vi "Get Tables.vi"(8 "error in (no error)":errorcluster, 10 "System Tables (F)":bool, 11 "MS Access in":refnum<class "MS Access.lvclass">) -> (0 "error out":errorcluster, 2 "Table Names":string[](array[string]), 3 "MS Access out":refnum<class "MS Access.lvclass">)   [LabVIEW 2020, in "MS Access.lvclass"]
uses:
  MS Access.lvclass
  ODBC/ADODB.lvclass
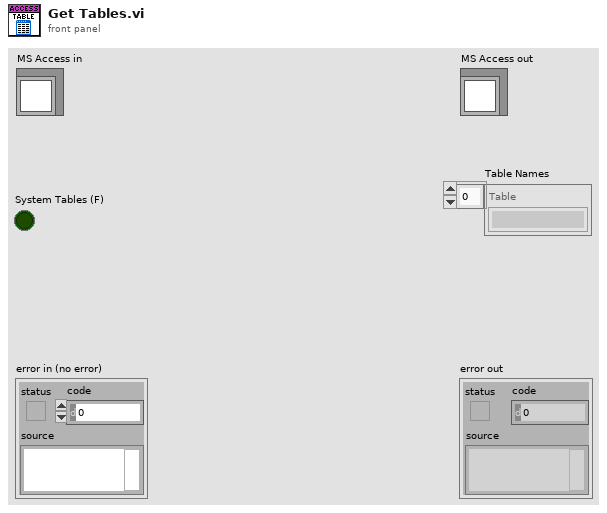
[diagram p1: front panel]
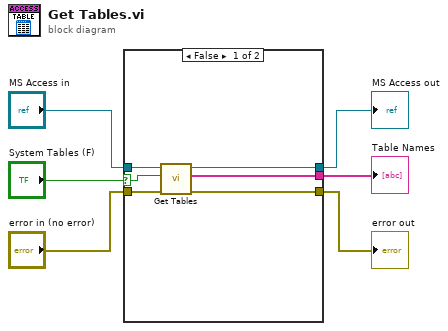
[diagram p0: block diagram]
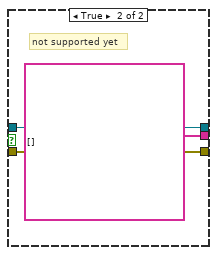
[diagram p2: hidden frame]
diagram:
  n1 = case shown="False" "System Tables (F)" {
    selector: "System Tables (F)" -> [w7 _]
    tunnel: [w12 w14] -> w6
    tunnel: [w11 string[] [] ("Table Names")] -> w5
    tunnel: [w10 w15] -> w4
    tunnel: "error in (no error)" -> [w9 w14]
    tunnel: "MS Access in" -> [w8 w15]
    frame False {
      n2 = call-parent "Get Tables.vi"("error in (no error)"=w9, "System Tables (F)"=w7, "ODBC in"=w8) -> ("error out"=w12:errorcluster, "Table Names"=w11:string[], "ODBC out"=w10:refnum<class "MS Access.lvclass">)  [unwired: 6 in]
    }
    frame True {
      # "not supported yet"
    }
  }
  "error out" <- w6
  "MS Access out" <- w4
  "Table Names" <- w5
